vi "Read Analogue.vi"(8 "error in (no error)":errorcluster, 11 "NI DMM in":refnum<class "NI DMM.lvclass">) -> (0 "error out":errorcluster, 2 "Waveforms":waveform(dbl)[](array[waveform]), 3 "NI DMM out":refnum<class "NI DMM.lvclass">)   [LabVIEW 2025, in "DMM.lvlib" / "NI DMM.lvclass"]
uses:
  NI DMM.lvclass
  C:/Users/Public/Documents/Sandia National Labs/TSS Plugin/Abstract Engine.lvlibp/Abstract Instrument/Abstract Instrument.lvclass
  NI DMM.lvclass/NI DMM.ctl
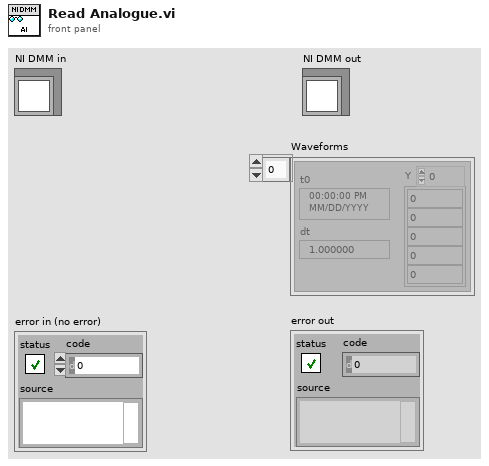
[diagram p1: front panel]
types:
  T1 = typedef "Abstract Engine.lvlibp/Abstract Instrument.lvclass/Channel.ctl" = cluster{"Alias":string, "DataType":enum16{"Anaolg Input", "Waveform"}, "Unit":enum16{"---", "V", "A", "Ohm", "Hz", "uF", "degC", "deg"}, "Upper limit":dbl, "Lower limit":dbl, "Measurement":variant}
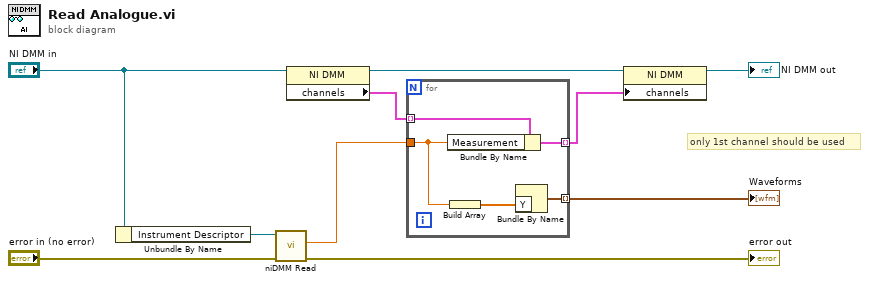
[diagram p0: block diagram]
diagram:
  # "only 1st channel should be used"
  n1 = Unbundle By Name("NI DMM in") -> ("Instrument Descriptor"=w9:refnum<k15>)
  n2 = call <instrlib>:"niDMM Read.vi"("error in (no error)"="error in (no error)", "instrument handle"=w9) -> ("error out"=→"error out":errorcluster, "Measurement"=w2:dbl)  [unwired: 1 in, 7 out]
  n3 = property class="NI DMM"(reference="NI DMM in") -> (reference out=w5:refnum<class "NI DMM.lvclass">, "channels"=w4:T1[])  [unwired: 1 in, 1 out]
  n4 = for {
    tunnel: w4 -> [w15] mode=indexing
    tunnel: [w14] -> w3 mode=indexing
    tunnel: w2 -> [w12]
    tunnel: [w11] -> w1 mode=indexing
    n5 = Bundle By Name(cluster=w15, "Measurement"=w12) -> (w14:T1)
    n6 = Build Array(w12) -> (w13:dbl[])
    n7 = Bundle By Name("Y"=w13) -> (w11:waveform(dbl))  [unwired: 1 in]
  }
  "Waveforms" <- w1
  n8 = property class="NI DMM"(reference=w5, "channels"=w3) -> (reference out=→"NI DMM out":refnum<class "NI DMM.lvclass">)  [unwired: 1 in, 1 out]
